vi "Delete file (Recycle Bin).vi"(8 "error in (no error)":errorcluster, 11 "Path":path) -> (0 "error out":errorcluster, 3 "Deleted path":path)   [LabVIEW 2011, in "COSYLib.lvlib"]
doc: "Delete a file, sending it to the Windows Recycle Bin (instead of deleting it permanently).\n\nNote: uses the .NET framework (Microsoft.VisualBasic assembly)."
uses:
  COSYLib.lvlib
  Microsoft.VisualBasic
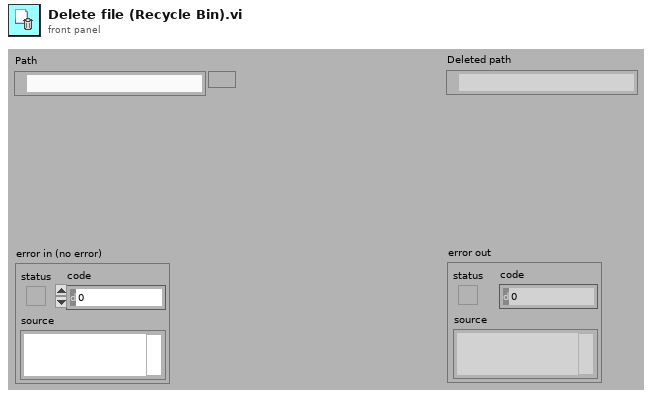
[diagram p1: front panel]
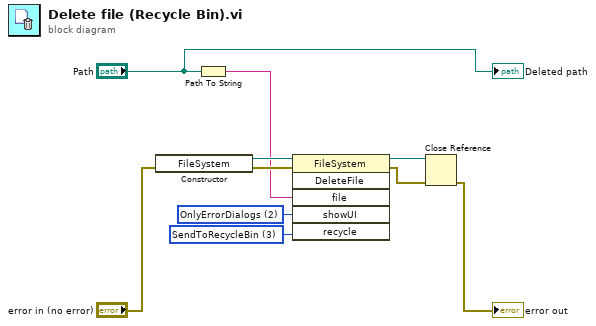
[diagram p0: block diagram]
diagram:
  w6 = 3 items=["DeletePermanently"=2, "SendToRecycleBin"=3] ("recycle")
  w7 = 2 items=["OnlyErrorDialogs"=2, "AllDialogs"=3] ("showUI")
  n1 = constructor class="FileSystem"(error in="error in (no error)") -> (reference out=w9:refnum<k24>, error out=w10:errorcluster)  [unwired: 2 in, 1 out]
  n2 = Path To String(path="Path") -> (string=w8:string)
  n3 = invoke class="FileSystem" method="DeleteFile"(reference=w9, error in=w10, "file"=w8, "showUI"=w7, "recycle"=w6) -> (reference out=w5:refnum<k24>, error out=w4:errorcluster)  [unwired: 1 in, 4 out]
  n4 = Close Reference(reference=w5, error in (no error)=w4) -> (error out=→"error out":errorcluster)
  "Deleted path" <- "Path"
